vi "Run Step.vi"(8 "error in (no error)":errorcluster, 9 "result allocation":T1, 10 "parameters":T1, 11 "Update Tag in":refnum<class "Update Tag.lvclass">) -> (0 "error out":errorcluster, 1 "results":T1, 2 "parameter allocation":T1, 3 "Update Tag out":refnum<class "Update Tag.lvclass">)   [LabVIEW 2015, in "Update Tag.lvclass"]
uses:
  Update Tag.lvclass
  <vilib>/NI/Tag Bus/table/data table.ctl
  classes/Step/Execution/StepState.ctl
  classes/Step/Execution/Step State Enum.ctl
  classes/Step/Execution/Step Flow Control.ctl
  Update Tag.lvclass/Update Tag.ctl
  <vilib>/NI/Tag Bus/table/data polymorphs/write one/write Double.vi
  <vilib>/NI/Tag Bus/table/data polymorphs/write one/write I32.vi
  <vilib>/NI/Tag Bus/table/data polymorphs/write one/write Boolean.vi
  <vilib>/NI/Tag Bus/table/data polymorphs/write one/write String.vi
  <vilib>/NI/Tag Bus/table/data polymorphs/write one/write Array of Boolean.vi
  <vilib>/NI/Tag Bus/table/data polymorphs/write one/write Array of Double.vi
  <vilib>/NI/Tag Bus/table/data polymorphs/write one/write Array of I32.vi
  <vilib>/NI/Tag Bus/table/data polymorphs/write one/write Array of String.vi
  <vilib>/NI/Tag Bus/table/data table.lvlib
  classes/Step/Execution/Step.lvclass
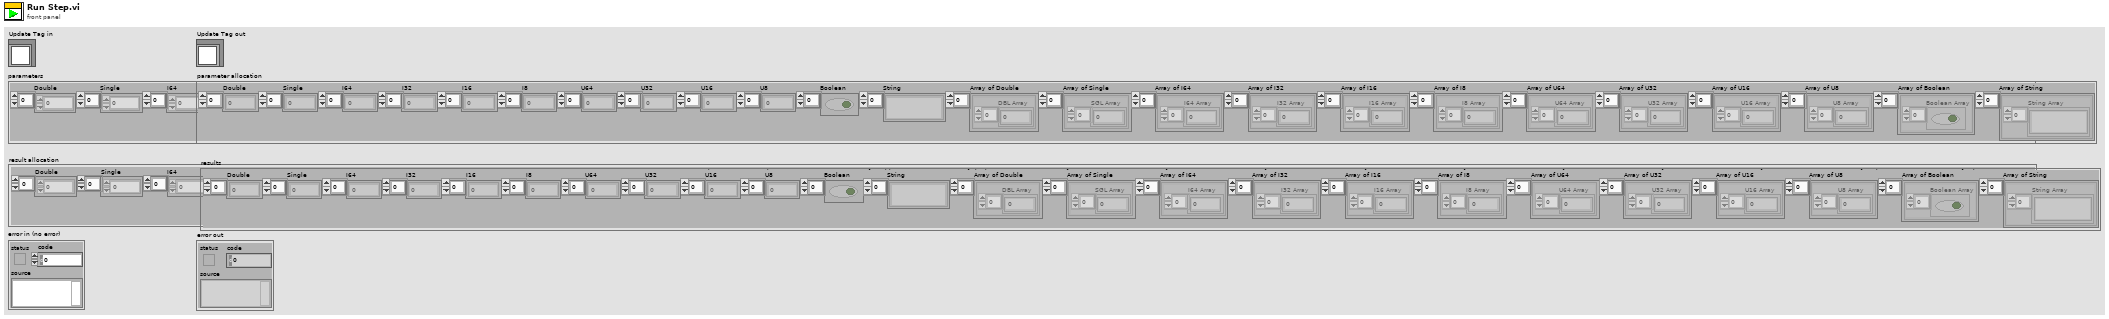
[diagram p1: front panel]
types:
  T1 = typedef "tag bus.lvlib/data table.lvlib/data table.ctl" = cluster{"Double":dbl[], "Single":sgl[], "I64":i64[], "I32":i32[], "I16":i16[], "I8":i8[], "U64":u64[], "U32":u32[], "U16":u16[], "U8":u8[], "Boolean":bool[], "String":string[], "Array of Double":cluster{"DBL Array":dbl[]}[], "Array of Single":cluster{"SGL Array":sgl[]}[], "Array of I64":cluster{"I64 Array":i64[]}[], "Array of I32":cluster{"I32 Array":i32[]}[], "Array of I16":cluster{"I16 Array":i16[]}[], "Array of I8":cluster{"I8 Array":i8[]}[], "Array of U64":cluster{"U64 Array":u64[]}[], "Array of U32":cluster{"U32 Array":u32[]}[], "Array of U16":cluster{"U16 Array":u16[]}[], "Array of U8":cluster{"U8 Array":u8[]}[], "Array of Boolean":cluster{"Boolean Array":bool[]}[], "Array of String":cluster{"String Array":string[]}[]}
  T2 = typedef "Step.lvclass/StepState.ctl" = cluster{"Step State":T3, "Flow Control":T4, "Jump Index":i32}
  T3 = typedef "Step.lvclass/Step State Enum.ctl" = enum16{"Start", "Skipped", "Completed", "Running", "Aborted"}
  T4 = typedef "Step.lvclass/Step Flow Control.ctl" = enum16{"Next Step", "Jump"}
  T5 = typedef "tag bus.lvlib/tag descriptor.lvclass/Data Type.ctl" = enum16{"Double", "Single", "I64", "I32", "I16", "I8", "U64", "U32", "U16", "U8", "Boolean", "String", "Array of Double", "Array of Single", "Array of I64", "Array of I32", "Array of I16", "Array of I8", "Array of U64", "Array of U32", "Array of U16", "Array of U8", "Array of Boolean", "Array of String"}
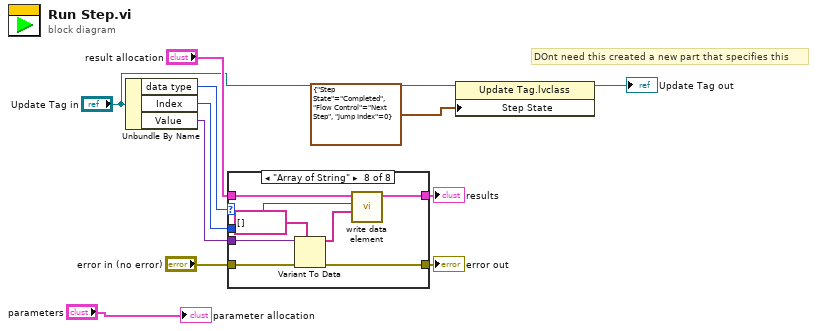
[diagram p0: block diagram]
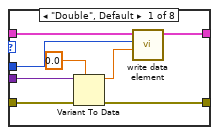
[diagram p2: hidden frame]
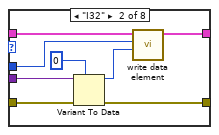
[diagram p3: hidden frame]
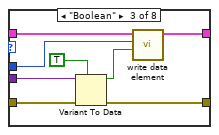
[diagram p4: hidden frame]
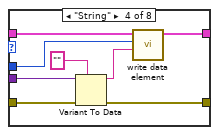
[diagram p5: hidden frame]
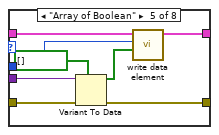
[diagram p6: hidden frame]
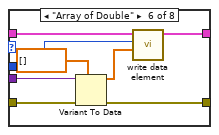
[diagram p7: hidden frame]
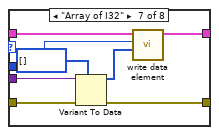
[diagram p8: hidden frame]
diagram:
  # "DOnt need this created a new part that specifies this"
  n1 = Unbundle By Name("Update Tag in") -> ("data type"=w11:T5, "Index"=w10:i32, "Value"=w8:variant)
  n2 = case shown="\"Array of String\"" w11 {
    tunnel: w10 -> [w18 w26 w34 w42 w50 w58 w66 w74]
    tunnel: "result allocation" -> [w19 w27 w35 w43 w51 w59 w67 w75]
    tunnel: w8 -> [w17 w25 w33 w41 w49 w57 w65 w73]
    tunnel: [w14 w22 w31 w39 w47 w55 w63 w71] -> w7
    tunnel: "error in (no error)" -> [w13 w21 w30 w38 w46 w54 w62 w70]
    tunnel: [w12 w20 w29 w37 w45 w53 w61 w69] -> w5
    frame "Double", Default {
      n3 = Variant To Data(error in=w13, type=0.0 ("value"), Variant=w17) -> (data=w15:dbl, error out=w12:errorcluster)
      n4 = call-poly <vilib>:"write data element.vi"("value"=w15, "index"=w18, "data table in"=w19) -> ("data table out"=w14:T1)  [unwired: 8 in]
    }
    frame "I32" {
      n5 = Variant To Data(error in=w21, type=0 ("value"), Variant=w25) -> (data=w23:i32, error out=w20:errorcluster)
      n6 = call-poly <vilib>:"write data element.vi"("value"=w23, "index"=w26, "data table in"=w27) -> ("data table out"=w22:T1)  [unwired: 8 in]
    }
    frame "Boolean" {
      n7 = Variant To Data(error in=w30, type=TRUE ("Completed"), Variant=w33) -> (data=w32:bool, error out=w29:errorcluster)
      n8 = call-poly <vilib>:"write data element.vi"("value"=w32, "index"=w34, "data table in"=w35) -> ("data table out"=w31:T1)  [unwired: 8 in]
    }
    frame "String" {
      n9 = Variant To Data(error in=w38, type="" ("Completed"), Variant=w41) -> (data=w40:string, error out=w37:errorcluster)
      n10 = call-poly <vilib>:"write data element.vi"("value"=w40, "index"=w42, "data table in"=w43) -> ("data table out"=w39:T1)  [unwired: 8 in]
    }
    frame "Array of Boolean" {
      n11 = Variant To Data(error in=w46, type=bool[] [] ("Completed"), Variant=w49) -> (data=w48:bool[], error out=w45:errorcluster)
      n12 = call-poly <vilib>:"write data element.vi"("value"=w48, "index"=w50, "data table in"=w51) -> ("data table out"=w47:T1)  [unwired: 8 in]
    }
    frame "Array of Double" {
      n13 = Variant To Data(error in=w54, type=dbl[] [] ("Completed"), Variant=w57) -> (data=w56:dbl[], error out=w53:errorcluster)
      n14 = call-poly <vilib>:"write data element.vi"("value"=w56, "index"=w58, "data table in"=w59) -> ("data table out"=w55:T1)  [unwired: 8 in]
    }
    frame "Array of I32" {
      n15 = Variant To Data(error in=w62, type=i32[] [] ("Completed"), Variant=w65) -> (data=w64:i32[], error out=w61:errorcluster)
      n16 = call-poly <vilib>:"write data element.vi"("value"=w64, "index"=w66, "data table in"=w67) -> ("data table out"=w63:T1)  [unwired: 8 in]
    }
    frame "Array of String" {
      n17 = Variant To Data(error in=w70, type=string[] [] ("Completed"), Variant=w73) -> (data=w72:string[], error out=w69:errorcluster)
      n18 = call-poly <vilib>:"write data element.vi"("value"=w72, "index"=w74, "data table in"=w75) -> ("data table out"=w71:T1)  [unwired: 8 in]
    }
  }
  "error out" <- w5
  "results" <- w7
  n19 = property class="Update Tag.lvclass"(reference="Update Tag in", "Step State"=T2 {"Step State"=enum."Completed", "Flow Control"=enum."Next Step", "Jump Index"=0}) -> (reference out=→"Update Tag out":refnum<class "Update Tag.lvclass">)  [unwired: 1 in, 1 out]
  "parameter allocation" <- "parameters"
